vi "xiC - Init.vi"(8 "error in (no error)":errorcluster, 11 "Attributes In":T1) -> (0 "error out":errorcluster, 3 "Attributes Out":T1)   [LabVIEW 2015]
uses:
  xiC - Attributes.ctl
  C:/GIT/Cameras3.x/Integrations/Labview/xiLib/xiLIB_32bit/xiLIB/xiCamLib/API/x86/xiApi.NET.dll
  xiLIB_32bit/xiLIB/xiCamLib/API/x86/xiApi.NET.dll
  xiC - TreeDisplayType.ctl
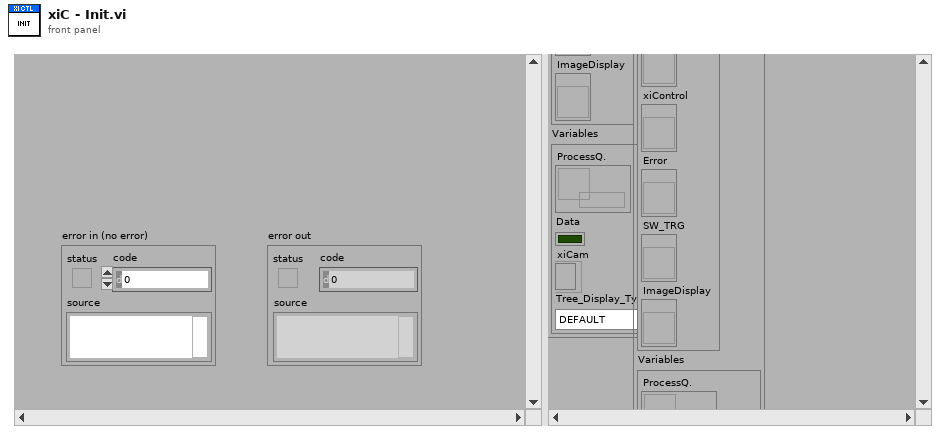
[diagram p1: front panel]
types:
  T1 = typedef "xiC - Attributes.ctl" = cluster{"Controls":cluster{"VI Ref.":refnum<vi>, "Tree":refnum<vi>, "Info":refnum<vi>, "PRMName":refnum<vi>, "xiControl":refnum<vi>, "Error":refnum<vi>, "SW_TRG":refnum<vi>, "ImageDisplay":refnum<vi>}, "Variables":cluster{"ProcessQ.":refnum<queue>, "Data":bool, "xiCam":refnum<k24>, "Tree_Display_Type":T2}}
  T2 = typedef "xiC - TreeDisplayType.ctl" = enum16{"DEFAULT", "HIDE_MAX_MIN"}
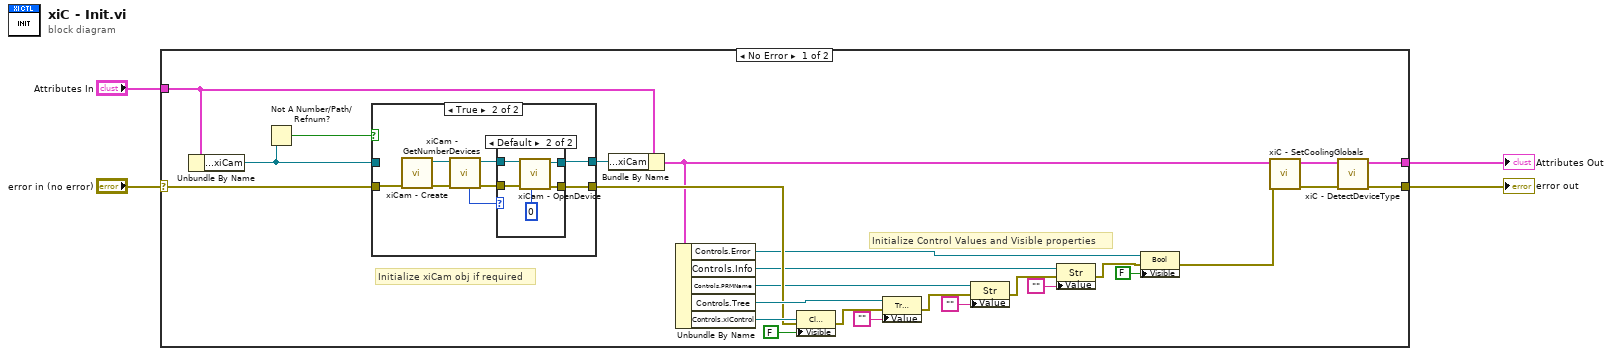
[diagram p0: block diagram]
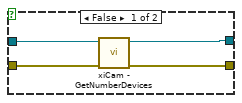
[diagram p2: hidden frame]
diagram:
  n1 = case shown="No Error" "error in (no error)" {
    selector: "error in (no error)" -> [w26 w51]
    tunnel: [w5 w51] -> w3
    tunnel: "Attributes In" -> [w28 w50]
    tunnel: [w7 w50] -> w1
    frame No Error {
      # "Initialize xiCam obj if required"
      # "Initialize Control Values and Visible properties"
      n2 = Unbundle By Name(w28) -> ("Variables.xiCam"=w29:refnum<k24>)
      n3 = Not A Number/Path/Refnum?(number/path/refnum=w29) -> (NaN/Path/Refnum?=w30:bool)
      n4 = case shown="True" w30 {
        tunnel: [w32 w38] -> w27
        tunnel: w29 -> [w34 _]
        tunnel: w26 -> [w33 w41]
        tunnel: [w31 w36] -> w21
        frame False {
          n5 = call "xiCam - GetNumberDevices.vi"("error in (no error)"=w33, "xiCam In"=w34) -> ("error out"=w31:errorcluster, "xiCam Out"=w32:refnum<k24>)  [unwired: 7 in, 1 out]
        }
        frame True {
          n6 = call "xiCam - Create.vi"("error in (no error)"=w41) -> ("error out"=w40:errorcluster, "new xiCam"=w42:refnum<k24>)  [unwired: 9 in]
          n7 = call "xiCam - GetNumberDevices.vi"("error in (no error)"=w40, "xiCam In"=w42) -> ("error out"=w37:errorcluster, "xiCam Out"=w39:refnum<k24>, "GetNumberDevices"=w35:i32)  [unwired: 7 in]
          n8 = case shown="Default" w35 {
            tunnel: w39 -> [w44 w49]
            tunnel: [w44 w48] -> w38
            tunnel: w37 -> [w43 w47]
            tunnel: [w43 w46] -> w36
            frame 0 {
            }
            frame Default {
              n9 = call "xiCam - OpenDevice.vi"("DevID"=0, "error in (no error)"=w47, "xiCam In"=w49) -> ("error out"=w46:errorcluster, "xiCam Out"=w48:refnum<k24>)  [unwired: 7 in]
            }
          }
        }
      }
      n10 = Bundle By Name(cluster=w28, "Variables.xiCam"=w27) -> (w10:T1)
      n11 = Unbundle By Name(w10) -> ("Controls.Error"=w12:refnum<vi>, "Controls.Info"=w15:refnum<vi>, "Controls.PRMName"=w18:refnum<vi>, "Controls.Tree"=w23:refnum<vi>, "Controls.xiControl"=w25:refnum<vi>)
      n12 = property class="Clust (strict)"(reference=w25, error in=w21, "Visible"=FALSE) -> (error out=w20:errorcluster)  [unwired: 1 out]
      n13 = property class="Tree (strict)"(reference=w23, error in=w20, "Value"="") -> (error out=w17:errorcluster)  [unwired: 1 out]
      n14 = property class="Str"(reference=w18, error in=w17, "Value"="") -> (error out=w14:errorcluster)  [unwired: 1 out]
      n15 = property class="Str"(reference=w15, error in=w14, "Value"="") -> (error out=w11:errorcluster)  [unwired: 1 out]
      n16 = property class="Bool"(reference=w12, error in=w11, "Visible"=FALSE) -> (error out=w9:errorcluster)  [unwired: 1 out]
      n17 = call "xiC - SetCoolingGlobals.vi"("error in (no error)"=w9, "Attributes In"=w10) -> ("error out"=w6:errorcluster, "Attributes Out"=w8:T1)  [unwired: 8 in]
      n18 = call "xiC - DetectDeviceType.vi"("error in (no error)"=w6, "Attributes In"=w8) -> ("error out"=w5:errorcluster, "Attributes Out"=w7:T1)  [unwired: 8 in]
    }
    frame Error {
    }
  }
  "error out" <- w3
  "Attributes Out" <- w1
